vi "UI_Elmt_Read(Label)-I32.vi"(8 "error in (no error)":errorcluster, 10 "Elmt Label":string, 11 "UI_Actor in":refnum<class "UI_Actor.lvclass">) -> (0 "error out":errorcluster, 1 "Found":bool, 2 "Value":i32, 3 "UI_Actor out":refnum<class "UI_Actor.lvclass">)   [LabVIEW 2020, in "UI_Actor.lvlib" / "UI_Actor.lvclass"]
doc: "Accès à un élément par son label.\n<b> NEVER USE IN FOR LOOP </b> \nLa ref est stockée au premier appel en fgv.\nLe VI doit etre dédié à un unique élement."
uses:
  UI_Actor.lvclass
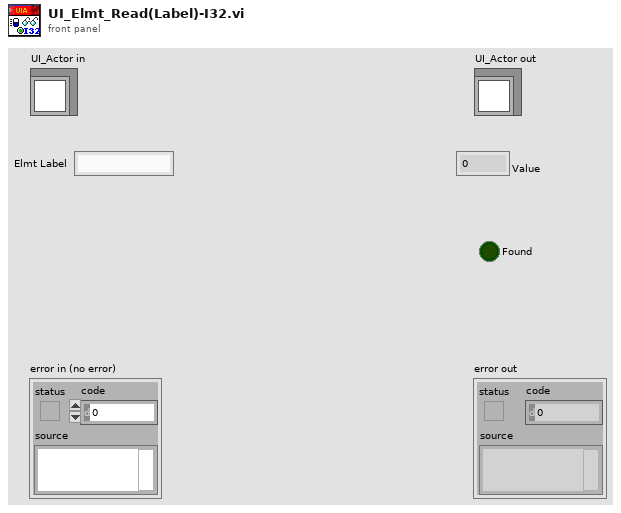
[diagram p1: front panel]
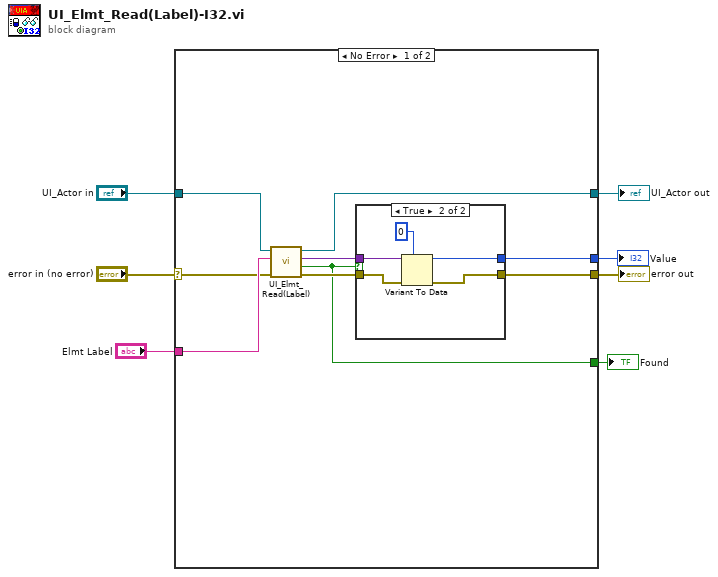
[diagram p0: block diagram]
diagram:
  n1 = case shown="No Error" "error in (no error)" {
    selector: "error in (no error)" -> [w14 w24]
    tunnel: [w10 w24] -> w6
    tunnel: [w13 w23] -> w4
    tunnel: "UI_Actor in" -> [w16 w23]
    tunnel: "Elmt Label" -> [w15 _]
    tunnel: [w9 _] -> w2
    tunnel: [w8 _] -> w1
    frame No Error {
      n2 = call "UI_Elmt_Read(Label).vi"("error in (no error)"=w14, "Elmt Label"=w15, "UI_Actor in"=w16) -> ("error out"=w11:errorcluster, "Found"=w8:bool, "Value"=w12:variant, "UI_Actor out"=w13:refnum<class "UI_Actor.lvclass">)  [unwired: 5 in]
      n3 = case shown="True" w8 {
        tunnel: w12 -> [_ w22]
        tunnel: w11 -> [w17 w21]
        tunnel: [w17 w20] -> w10
        tunnel: [_ w18] -> w9
        frame False {
        }
        frame True {
          n4 = Variant To Data(error in=w21, type=0, Variant=w22) -> (data=w18:i32, error out=w20:errorcluster)
        }
      }
    }
    frame Error {
    }
  }
  "error out" <- w6
  "UI_Actor out" <- w4
  "Value" <- w2
  "Found" <- w1
